vi "Request_NIPath.vi"(8 "error in (no error)":errorcluster, 11 "Dest_NI_NIPath in":refnum<class "Dest_NI_NIPath.lvclass">) -> (0 "error out":errorcluster, 3 "Dest_NI_NIPath out":refnum<class "Dest_NI_NIPath.lvclass">)   [LabVIEW 2020, in "Dest_NI_NIPath.lvclass"]
uses:
  <vilib>/AppBuilder/IB_Classes/Dest_NI_NIPath/Dest_NI_NIPath.lvclass
  <vilib>/AppBuilder/IB_Classes/Dest_NI_NIPath/Dest_NI_NIPath.lvclass/Dest_NI_NIPath.ctl
  AppLibs/distkit/MDF/NI_MDF.lvlib
  <vilib>/AppBuilder/IB_Classes/Destination/IB_Destination.lvclass
  e:/builds/penguin/labview/branches/2020/dev/dist/vi.lib/AppBuilder/IB_Classes/Destination/niLabel/niLabel.lvclass
  e:/builds/penguin/labview/branches/2020/dev/dist/vi.lib/AppBuilder/IB_Classes/Destination/IB_Destination.lvclass
  e:/builds/penguin/labview/branches/2020/dev/dist/vi.lib/AppBuilder/IB_Classes/Dest_NI_NIPath/Dest_NI_NIPath.lvclass
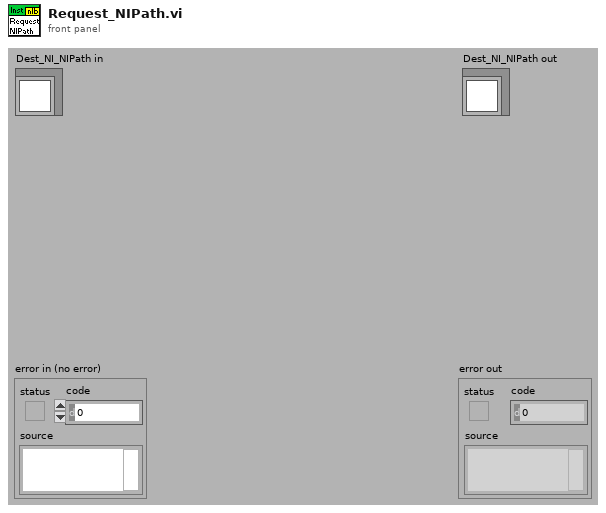
[diagram p1: front panel]
types:
  T1 = typedef "IB_Destination.ctl" = cluster{"name":string, "unlock":bool, "parentTag":string, "destTag":string, "eng_installPath":string}
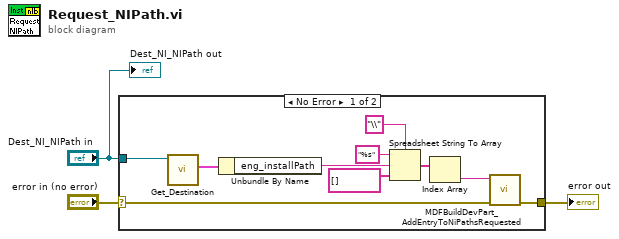
[diagram p0: block diagram]
diagram:
  n1 = case shown="No Error" "error in (no error)" {
    selector: "error in (no error)" -> [w10 w14]
    tunnel: [w13 w14] -> w3
    tunnel: "Dest_NI_NIPath in" -> [w12 _]
    frame No Error {
      n2 = call <vilib>:"Get_Destination.vi"("IB_Destination in"=w12) -> ("data"=w11:T1)  [unwired: 8 in, 2 out]
      n3 = Unbundle By Name(w11) -> ("eng_installPath"=w5:string)
      n4 = Spreadsheet String To Array(delimiter (Tab)="\\", format string="%s", spreadsheet string=w5, array type (2D Dbl)=string[] []) -> (array=w6:string[])
      n5 = Index Array(array=w6) -> (element=w4:string)  [unwired: 1 in]
      n6 = call "MDFBuildDevPart_AddEntryToNiPathsRequested.vi"("error in (no error)"=w10, "NI Path Name"=w4) -> ("error out"=w13:errorcluster)  [unwired: 9 out]
    }
    frame Error {
    }
  }
  "error out" <- w3
  "Dest_NI_NIPath out" <- "Dest_NI_NIPath in"
